vi "backupauto.vi"   [LabVIEW 2014, in "Janga.lvrbt"]
uses:
  Janga.lvrbt
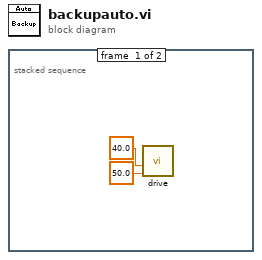
[diagram p0: block diagram]
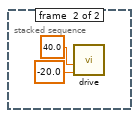
[diagram p2: hidden frame]
diagram:
  n1 = stacked-sequence {
    frame #0 {
      n2 = call "drive.vi"("Speed"=50.0, "Distance (cm)"=40.0) -> ()  [unwired: 10 in]
    }
    frame #1 {
      n3 = call "drive.vi"("Speed"=-20.0, "Distance (cm)"=40.0) -> ()  [unwired: 10 in]
    }
  }
